vi "raw_to_calibrated-array.vi"(5 "tag_names []":string[](array[string]), 7 "runtime":variant, 8 "error in (no error)":errorcluster, 11 "value in":dbl[](array[numeric])) -> (0 "error out":errorcluster, 3 "value out":dbl[](array[numeric]))   [LabVIEW 2015, in "lv-calibration.lvlib"]
uses:
  lv-calibration.lvlib
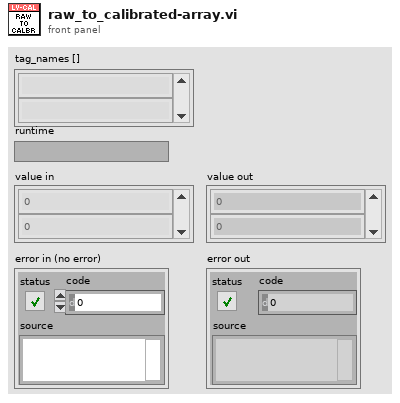
[diagram p1: front panel]
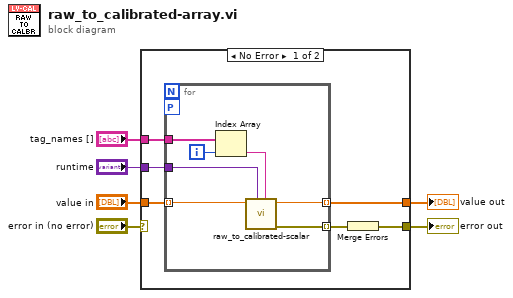
[diagram p0: block diagram]
diagram:
  n1 = case shown="No Error" "error in (no error)" {
    selector: "error in (no error)" -> [_ w20]
    tunnel: "value in" -> [w11 _]
    tunnel: [w7 w20] -> w5
    tunnel: "runtime" -> [w9 _]
    tunnel: "tag_names []" -> [w8 _]
    tunnel: [w10 _] -> w1
    frame No Error {
      n2 = for {
        tunnel: w11 -> [w18] mode=indexing
        tunnel: [w17] -> w10 mode=indexing
        tunnel: w9 -> [w16]
        tunnel: w8 -> [w15]
        tunnel: [w19] -> w12 mode=indexing
        workers-P: _ -> [_]
        i -> [w13]
        n3 = Index Array(array=w15, index=w13) -> (element=w14:string)
        n4 = call "raw_to_calibrated-scalar.vi"("tag_name"=w14, "runtime"=w16, "value in"=w18) -> ("error out"=w19:errorcluster, "value out"=w17:dbl)  [unwired: 7 in]
      }
      n5 = Merge Errors(w12) -> (w7:errorcluster)
    }
    frame Error {
    }
  }
  "error out" <- w5
  "value out" <- w1
